vi "Attack Array.vi"(4 "Y":i32, 6 "X":i32, 8 "error in":errorcluster, 9 "add attack":bool, 10 "Direction":T1, 11 "Round":i32) -> (0 "error out":errorcluster, 2 "attack array":bool[][](array[boolean]), 3 "Round out":i32)   [LabVIEW 2017, in "Uno.lvclass"]
uses:
  Uno.lvclass
  Type Defs/Direction Enum.ctl
  SubVIs/Read-Only Globals.vi
  SubVIs/Globals (private).vi
  Square/Square.lvclass
  Type Defs/SB Type Defs.lvlib
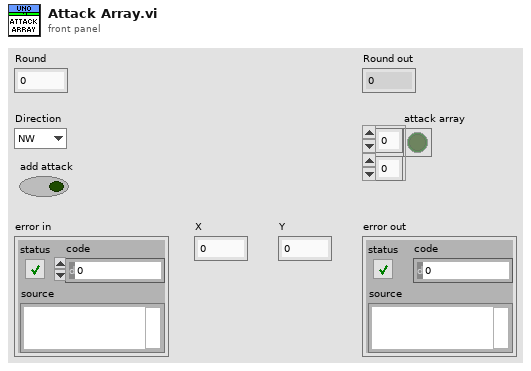
[diagram p1: front panel]
types:
  T1 = typedef "SB Type Defs.lvlib/Direction Enum.ctl" = enum16{"NW", "N", "NE", "E", "SE", "S", "SW", "W"}
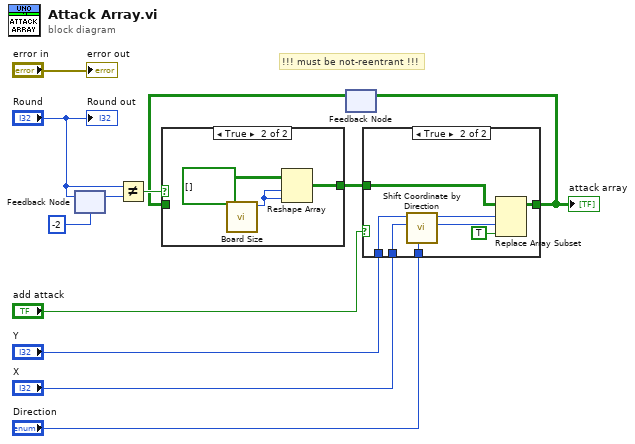
[diagram p0: block diagram]
diagram:
  # "!!! must be not-reentrant !!!"
  n1 = feedback-in #1("Round") -> ()
  n2 = feedback #1(-2 ("Round")) -> (w10:i32)
  n3 = Not Equal?(x="Round", y=w10) -> (x != y?=w9:bool)
  n4 = feedback #2() -> (w8:bool[][])  [unwired: 1 in]
  n5 = case shown="True" w9 {
    tunnel: w8 -> [w13 _]
    tunnel: [w13 w14] -> w7
    frame False {
    }
    frame True {
      n6 = call "Board Size.vi"() -> ("Board Size"=w16:i32)  [unwired: 11 in]
      n7 = Reshape Array(bool[][] [] ("boolean array"), w16, w16) -> (w14:bool[][])
    }
  }
  n8 = case shown="True" "add attack" {
    tunnel: w7 -> [w17 w25]
    tunnel: [w17 w24] -> w5
    tunnel: "Y" -> [_ w20]
    tunnel: "X" -> [_ w19]
    tunnel: "Direction" -> [_ w18]
    frame False {
    }
    frame True {
      n9 = call "Shift Coordinate by Direction.vi"("Direction"=w18, "X in"=w19, "Y in"=w20) -> ("X out"=w21:i32, "Y out"=w22:i32)  [unwired: 7 in]
      n10 = Replace Array Subset(array=w25, new element=TRUE ("new element/subarray"), index (row)=w22, index (col)=w21) -> (w24:bool[][])
    }
  }
  "attack array" <- w5
  n11 = feedback-in #2(w5) -> ()
  "error out" <- "error in"
  "Round out" <- "Round"
